vi "Y_Jog_Plus.vi"(11 "Jog Y Up":bool) -> (3 "Final Y":sgl)   [LabVIEW 2013]
panel:
  in  "MG17Motor 3":refnum<k7>(container)
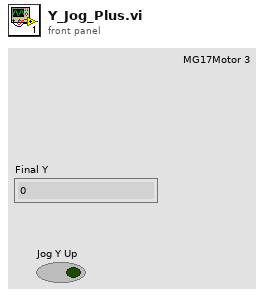
[diagram p1: front panel]
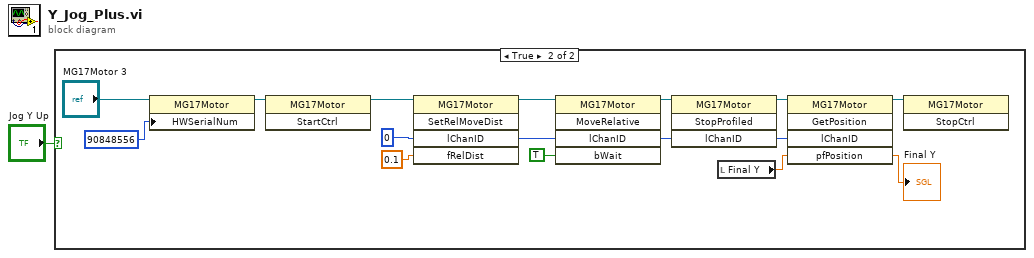
[diagram p0: block diagram]
diagram:
  n1 = case shown="True" "Jog Y Up" {
    frame False {
    }
    frame True {
      n2 = property class="MG17Motor"(reference="MG17Motor 3", "HWSerialNum"=90848556 ("lChanID")) -> (reference out=w16:refnum<k7>)  [unwired: 1 in, 1 out]
      n3 = invoke class="MG17Motor" method="StartCtrl"(reference=w16) -> (reference out=w2:refnum<k7>)  [unwired: 2 in, 2 out]
      n4 = invoke class="MG17Motor" method="SetRelMoveDist"(reference=w2, "lChanID"=0, "fRelDist"=0.1) -> (reference out=w7:refnum<k7>, "lChanID"=w8:i32)  [unwired: 2 in, 3 out]
      n5 = invoke class="MG17Motor" method="MoveRelative"(reference=w7, "lChanID"=w8, "bWait"=TRUE) -> (reference out=w9:refnum<k7>, "lChanID"=w10:i32)  [unwired: 2 in, 3 out]
      n6 = invoke class="MG17Motor" method="StopProfiled"(reference=w9, "lChanID"=w10) -> (reference out=w13:refnum<k7>, "lChanID"=w11:i32)  [unwired: 2 in, 2 out]
      n7 = local read "Final Y"() -> (w14:sgl)
      n8 = invoke class="MG17Motor" method="GetPosition"(reference=w13, "lChanID"=w11, "pfPosition"=w14) -> (reference out=w12:refnum<k7>, "pfPosition"=→"Final Y":sgl)  [unwired: 2 in, 3 out]
      n9 = invoke class="MG17Motor" method="StopCtrl"(reference=w12) -> ()  [unwired: 2 in, 3 out]
    }
  }
